vi "TDK_LoadCMD.vi"() -> (3 "PowerSupplyCMD":T1)   [LabVIEW 2018]
uses:
  Def Ctrl/PowerSupplyCMD.ctl
  Def Ctrl/CMD_String.ctl
  Def Ctrl/PowerInf.ctl
  Def Ctrl/TDK Type.ctl
  Def Ctrl/CMD Type.ctl
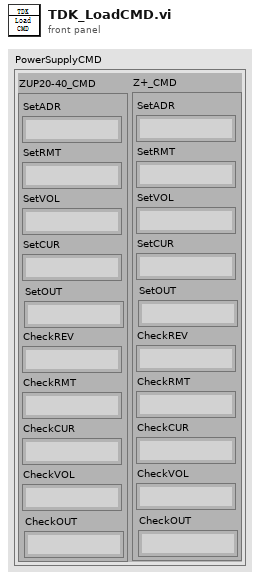
[diagram p1: front panel]
types:
  T1 = typedef "PowerSupplyCMD.ctl" = cluster{"ZUP20-40_CMD":T2, "Z+_CMD":T2}
  T2 = typedef "CMD_String.ctl" = cluster{"SetADR":string, "SetRMT":string, "SetVOL":string, "SetCUR":string, "SetOUT":string, "CheckREV":string, "CheckRMT":string, "CheckCUR":string, "CheckVOL":string, "CheckOUT":string}
  T3 = typedef "PowerInf.ctl" = cluster{"TDK Type":T4, "CMD Type":T5, "CMD String":string}
  T4 = typedef "TDK Type.ctl" = enum16{"Default", "ZUP20-40", "Z+"}
  T5 = typedef "CMD Type.ctl" = enum16{"Default", "SetADR", "SetRMT", "SetVOL", "SetCUR", "SetOUT", "CheckREV", "CheckRMT", "CheckVOL", "CkeckCUR", "CheckOUT"}
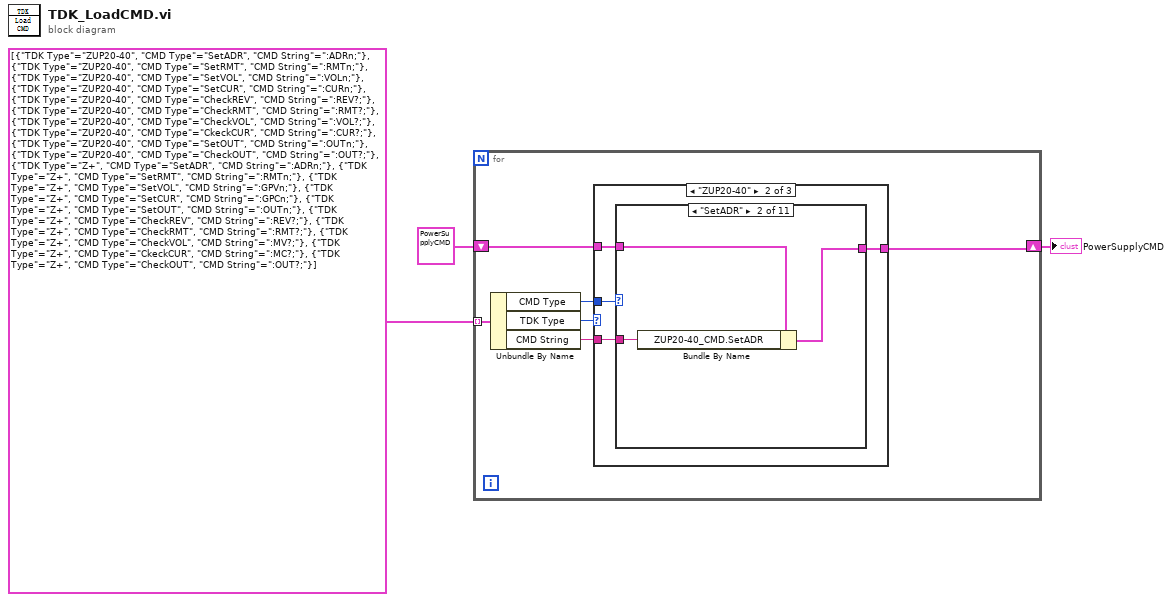
[diagram p0: block diagram]
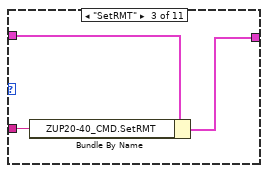
[diagram p4: hidden frame]
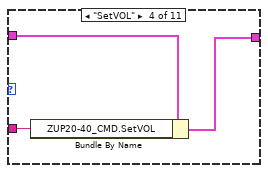
[diagram p5: hidden frame]
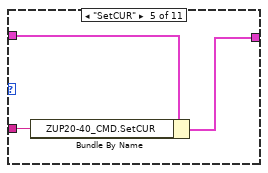
[diagram p6: hidden frame]
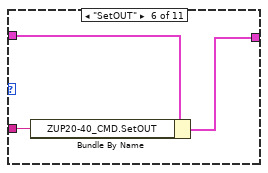
[diagram p7: hidden frame]
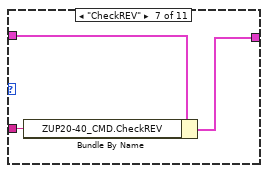
[diagram p8: hidden frame]
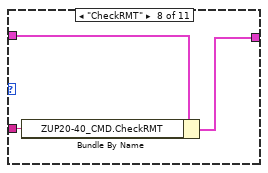
[diagram p9: hidden frame]
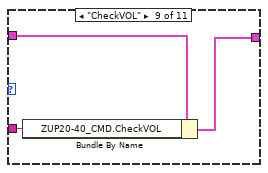
[diagram p10: hidden frame]
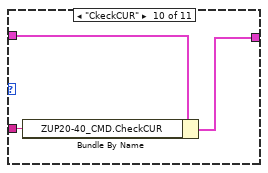
[diagram p11: hidden frame]
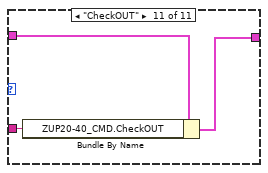
[diagram p12: hidden frame]
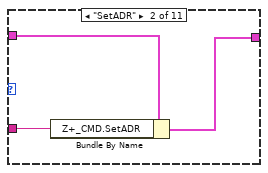
[diagram p14: hidden frame]
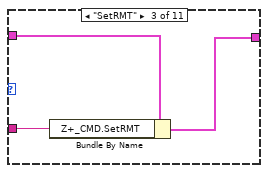
[diagram p15: hidden frame]
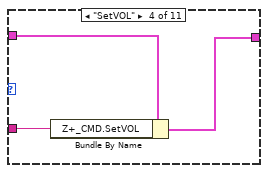
[diagram p16: hidden frame]
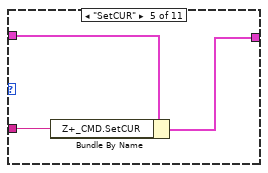
[diagram p17: hidden frame]
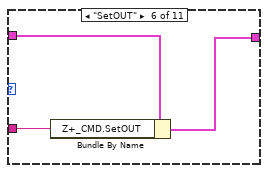
[diagram p18: hidden frame]
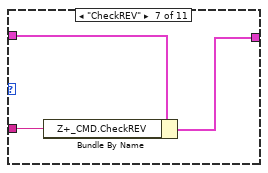
[diagram p19: hidden frame]
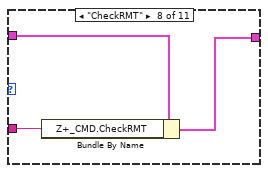
[diagram p20: hidden frame]
diagram:
  n1 = for {
    tunnel: T3[] [{"TDK Type"=enum."ZUP20-40", "CMD Type"=enum."SetADR", "CMD String"=":ADRn;"}, {"TDK Type"=enum."ZUP20-40", "CMD Type"=enum."SetRMT", "CMD String"=":RMTn;"}, {"TDK Type"=enum."ZUP20-40", "CMD Type"=enum."SetVOL", "CMD String"=":VOLn;"}, {"TDK Type"=enum."ZUP20-40", "CMD Type"=enum."SetCUR", "CMD String"=":CURn;"}, {"TDK Type"=enum."ZUP20-40", "CMD Type"=enum."CheckREV", "CMD String"=":REV?;"}, {"TDK Type"=enum."ZUP20-40", "CMD Type"=enum."CheckRMT", "CMD String"=":RMT?;"}, {"TDK Type"=enum."ZUP20-40", "CMD Type"=enum."CheckVOL", "CMD String"=":VOL?;"}, {"TDK Type"=enum."ZUP20-40", "CMD Type"=enum."CkeckCUR", "CMD String"=":CUR?;"}, {"TDK Type"=enum."ZUP20-40", "CMD Type"=enum."SetOUT", "CMD String"=":OUTn;"}, {"TDK Type"=enum."ZUP20-40", "CMD Type"=enum."CheckOUT", "CMD String"=":OUT?;"}, {"TDK Type"=enum."Z+", "CMD Type"=enum."SetADR", "CMD String"=":ADRn;"}, {"TDK Type"=enum."Z+", "CMD Type"=enum."SetRMT", "CMD String"=":RMTn;"}, {"TDK Type"=enum."Z+", "CMD Type"=enum."SetVOL", "CMD String"=":GPVn;"}, {"TDK Type"=enum."Z+", "CMD Type"=enum."SetCUR", "CMD String"=":GPCn;"}, {"TDK Type"=enum."Z+", "CMD Type"=enum."SetOUT", "CMD String"=":OUTn;"}, {"TDK Type"=enum."Z+", "CMD Type"=enum."CheckREV", "CMD String"=":REV?;"}, {"TDK Type"=enum."Z+", "CMD Type"=enum."CheckRMT", "CMD String"=":RMT?;"}, {"TDK Type"=enum."Z+", "CMD Type"=enum."CheckVOL", "CMD String"=":MV?;"}, {"TDK Type"=enum."Z+", "CMD Type"=enum."CkeckCUR", "CMD String"=":MC?;"}, {"TDK Type"=enum."Z+", "CMD Type"=enum."CheckOUT", "CMD String"=":OUT?;"}] -> [w8] mode=indexing
    shift-right: [w4] -> w1
    shift-left: T1 {"ZUP20-40_CMD"={"SetADR"="", "SetRMT"="", "SetVOL"="", "SetCUR"="", "SetOUT"="", "CheckREV"="", "CheckRMT"="", "CheckCUR"="", "CheckVOL"="", "CheckOUT"=""}, "Z+_CMD"={"SetADR"="", "SetRMT"="", "SetVOL"="", "SetCUR"="", "SetOUT"="", "CheckREV"="", "CheckRMT"="", "CheckCUR"="", "CheckVOL"="", "CheckOUT"=""}} ("PowerSupplyCMD") -> [w6]
    n2 = Unbundle By Name(w8) -> ("CMD Type"=w7:T5, "TDK Type"=w9:T4, "CMD String"=w5:string)
    n3 = case shown="\"ZUP20-40\"" w9 {
      tunnel: w7 -> [_ w14 w49]
      tunnel: w6 -> [w10 w13 w48]
      tunnel: w5 -> [_ w12 w47]
      tunnel: [w10 w11 w46] -> w4
      frame "Default", Default {
      }
      frame "ZUP20-40" {
        n4 = case shown="\"SetADR\"" w14 {
          tunnel: w13 -> [w15 w18 w21 w24 w27 w30 w33 w36 w39 w42 w45]
          tunnel: w12 -> [_ w17 w20 w23 w26 w29 w32 w35 w38 w41 w44]
          tunnel: [w15 w16 w19 w22 w25 w28 w31 w34 w37 w40 w43] -> w11
          frame "Default", Default {
          }
          frame "SetADR" {
            n5 = Bundle By Name(cluster=w18, "ZUP20-40_CMD.SetADR"=w17) -> (w16:T1)
          }
          frame "SetRMT" {
            n6 = Bundle By Name(cluster=w21, "ZUP20-40_CMD.SetRMT"=w20) -> (w19:T1)
          }
          frame "SetVOL" {
            n7 = Bundle By Name(cluster=w24, "ZUP20-40_CMD.SetVOL"=w23) -> (w22:T1)
          }
          frame "SetCUR" {
            n8 = Bundle By Name(cluster=w27, "ZUP20-40_CMD.SetCUR"=w26) -> (w25:T1)
          }
          frame "SetOUT" {
            n9 = Bundle By Name(cluster=w30, "ZUP20-40_CMD.SetOUT"=w29) -> (w28:T1)
          }
          frame "CheckREV" {
            n10 = Bundle By Name(cluster=w33, "ZUP20-40_CMD.CheckREV"=w32) -> (w31:T1)
          }
          frame "CheckRMT" {
            n11 = Bundle By Name(cluster=w36, "ZUP20-40_CMD.CheckRMT"=w35) -> (w34:T1)
          }
          frame "CheckVOL" {
            n12 = Bundle By Name(cluster=w39, "ZUP20-40_CMD.CheckVOL"=w38) -> (w37:T1)
          }
          frame "CkeckCUR" {
            n13 = Bundle By Name(cluster=w42, "ZUP20-40_CMD.CheckCUR"=w41) -> (w40:T1)
          }
          frame "CheckOUT" {
            n14 = Bundle By Name(cluster=w45, "ZUP20-40_CMD.CheckOUT"=w44) -> (w43:T1)
          }
        }
      }
      frame "Z+" {
        n15 = case shown="\"Default\", 默认" w49 {
          tunnel: w48 -> [w50 w53 w56 w59 w62 w65 w68 w71 w74 w77 w80]
          tunnel: w47 -> [_ w52 w55 w58 w61 w64 w67 w70 w73 w76 w79]
          tunnel: [w50 w51 w54 w57 w60 w63 w66 w69 w72 w75 w78] -> w46
          frame "Default", Default {
          }
          frame "SetADR" {
            n16 = Bundle By Name(cluster=w53, "Z+_CMD.SetADR"=w52) -> (w51:T1)
          }
          frame "SetRMT" {
            n17 = Bundle By Name(cluster=w56, "Z+_CMD.SetRMT"=w55) -> (w54:T1)
          }
          frame "SetVOL" {
            n18 = Bundle By Name(cluster=w59, "Z+_CMD.SetVOL"=w58) -> (w57:T1)
          }
          frame "SetCUR" {
            n19 = Bundle By Name(cluster=w62, "Z+_CMD.SetCUR"=w61) -> (w60:T1)
          }
          frame "SetOUT" {
            n20 = Bundle By Name(cluster=w65, "Z+_CMD.SetOUT"=w64) -> (w63:T1)
          }
          frame "CheckREV" {
            n21 = Bundle By Name(cluster=w68, "Z+_CMD.CheckREV"=w67) -> (w66:T1)
          }
          frame "CheckRMT" {
            n22 = Bundle By Name(cluster=w71, "Z+_CMD.CheckRMT"=w70) -> (w69:T1)
          }
          frame "CheckVOL" {
            n23 = Bundle By Name(cluster=w74, "Z+_CMD.CheckVOL"=w73) -> (w72:T1)
          }
          frame "CkeckCUR" {
            n24 = Bundle By Name(cluster=w77, "Z+_CMD.CheckCUR"=w76) -> (w75:T1)
          }
          frame "CheckOUT" {
            n25 = Bundle By Name(cluster=w80, "Z+_CMD.CheckOUT"=w79) -> (w78:T1)
          }
        }
      }
    }
  }
  "PowerSupplyCMD" <- w1
